vi "Write Allow Undefined Names.vi"(8 "error in (no error)":errorcluster, 10 "AllowUndefNames":bool, 11 "IVILogicalName.lvclass in":refnum<class "IVILogicalName.lvclass">) -> (0 "error out":errorcluster, 3 "IVILogicalName.lvclass out":refnum<class "IVILogicalName.lvclass">)   [LabVIEW 2015, in "IVILogicalName.lvclass"]
uses:
  IVILogicalName.lvclass
  IVILogicalName.lvclass/IVILogicalName.ctl
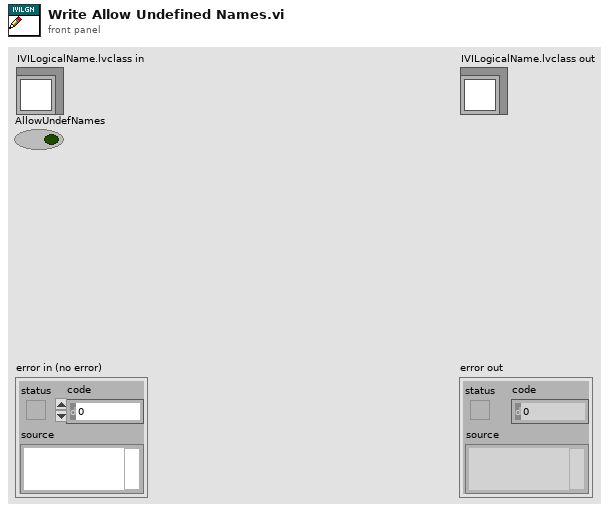
[diagram p1: front panel]
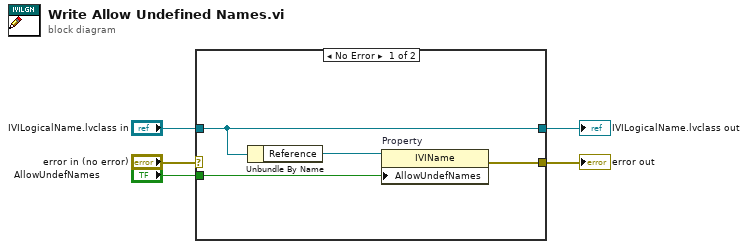
[diagram p0: block diagram]
diagram:
  n1 = case shown="No Error" "error in (no error)" {
    selector: "error in (no error)" -> [_ w11]
    tunnel: [w9 w11] -> w4
    tunnel: [w7 w10] -> w2
    tunnel: "IVILogicalName.lvclass in" -> [w7 w10]
    tunnel: "AllowUndefNames" -> [w8 _]
    frame No Error {
      n2 = Unbundle By Name(w7) -> ("Reference"=w6:refnum<vi>)
      n3 = property on="Property" class="IVIName"(reference=w6, "AllowUndefNames"=w8) -> (error out=w9:errorcluster)  [unwired: 1 in, 1 out]
    }
    frame Error {
    }
  }
  "error out" <- w4
  "IVILogicalName.lvclass out" <- w2
